vi "Read Version Text.vi"(8 "error in (no error)":errorcluster, 11 "Package Details in":refnum<class "Package Version.lvclass">) -> (0 "error out":errorcluster, 2 "Version Text":string, 3 "Package Details out":refnum<class "Package Version.lvclass">)   [LabVIEW 2016, in "Packages.lvlib" / "Package Version.lvclass"]
uses:
  Package Version.lvclass
  Package Version.lvclass/Package Version.ctl
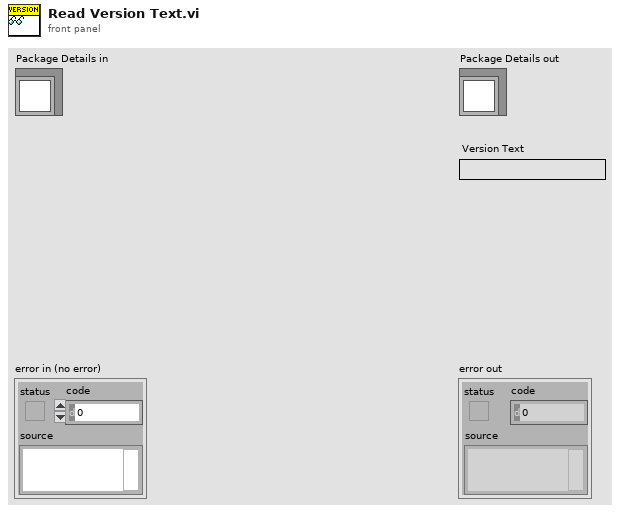
[diagram p1: front panel]
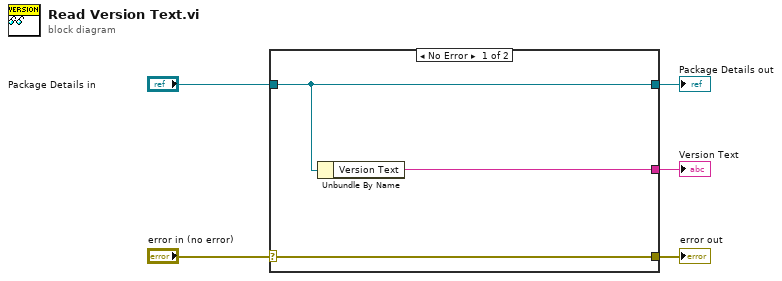
[diagram p0: block diagram]
diagram:
  n1 = case shown="No Error" "error in (no error)" {
    selector: "error in (no error)" -> [w8 w9]
    tunnel: [w8 w9] -> w4
    tunnel: [w7 w10] -> w2
    tunnel: "Package Details in" -> [w7 w10]
    tunnel: [w6 _] -> w1
    frame No Error {
      n2 = Unbundle By Name(w7) -> ("Version Text"=w6:string)
    }
    frame Error {
    }
  }
  "error out" <- w4
  "Package Details out" <- w2
  "Version Text" <- w1
